vi "Write daemon error.vi"(8 "error in (no error)":errorcluster, 10 "daemon error":errorcluster, 11 "Network Slave in":refnum<class "Network Slave.lvclass">) -> (0 "error out":errorcluster, 3 "Network Slave out":refnum<class "Network Slave.lvclass">)   [LabVIEW 2012, in "Network Slave.lvclass"]
uses:
  Network Slave.lvclass
  Network Slave.lvclass/Network Slave.ctl
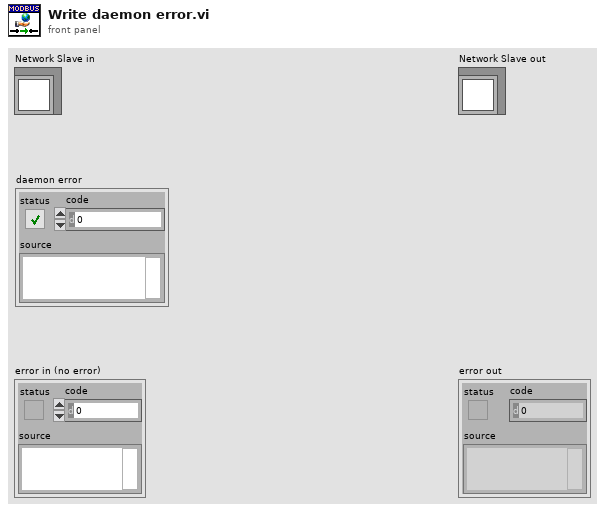
[diagram p1: front panel]
types:
  T1 = typedef "Network Slave.lvclass/daemon status cluster.ctl" = cluster{"error":errorcluster, "status":T2}
  T2 = typedef "Network Slave.lvclass/daemon status.ctl" = enum16{"Not Started", "Running", "Error", "Stopped"}
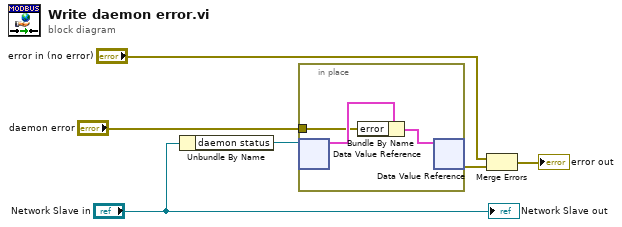
[diagram p0: block diagram]
diagram:
  n1 = Unbundle By Name("Network Slave in") -> ("daemon status"=w5:refnum<data-value>)
  n2 = in-place {
    in-place-border: "daemon error" -> [w7]
    n3 = in-place-dvr #1(w5) -> (w9:T1)  [unwired: 1 out]
    n4 = Bundle By Name(cluster=w9, "error"=w7) -> (w8:T1)
    n5 = in-place-dvr #1(w8) -> (w6:errorcluster)  [unwired: 1 out]
  }
  n6 = Merge Errors("error in (no error)", w6) -> (→"error out":errorcluster)
  "Network Slave out" <- "Network Slave in"
